vi "PS 180 Comm.vi"(2 "error in (no error)":errorcluster, 3 "?":string, 4 "VISA session":refnum<visa-resource-name>) -> (0 "error out":errorcluster, 1 "?":string)   [LabVIEW 2019]
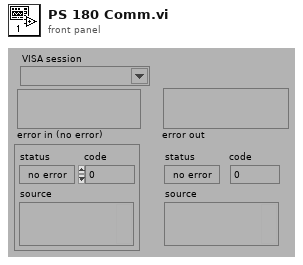
[diagram p1: front panel]
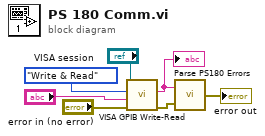
[diagram p0: block diagram]
diagram:
  n1 = call "VISA GPIB Write-Read.vi"("error in (no error)"="error in (no error)", "Command"="?", "Action"=enum16{"Write", "Read", "Write & Read"}."Write & Read", "VISA resource name"="VISA session") -> ("error out"=w6:errorcluster, "String Returned"=w5:string)  [unwired: 4 in, 2 out]
  "?" <- w5
  n2 = call "Parse PS180 Errors.vi"("error in (no error)"=w6, "PS 180 String"=w5) -> ("error out"=→"error out":errorcluster)
